vi "Update Room From Server.vi"(8 "error in":errorcluster, 11 "Room Array":refnum<class "Room.lvclass">[](array[class])) -> (0 "error out":errorcluster, 3 "Room Array Out":refnum<class "Room.lvclass">[](array[class]))   [LabVIEW 2015]
uses:
  LVClasses/Room/Room.lvclass
  LVRestAPI/TypeDef/GetRoomCommands.ctl
  LVClasses/Room/Room.lvclass/Room.ctl
  LVRestAPI/RestApi.lvlib
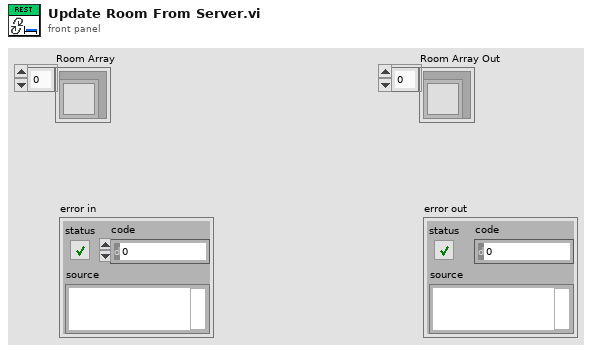
[diagram p1: front panel]
types:
  T1 = typedef "RestApi.lvlib/GetRoomCommands.ctl" = enum16{"ReadRoom", "ReadFlag", "ReadFlagState", "ReadFlagColor", "ReadBedVacant", "ReadPersonnel", "ReadRequests", "ReadBeaconID", "ReadBedURL", "ReadRoomsNumbers"}
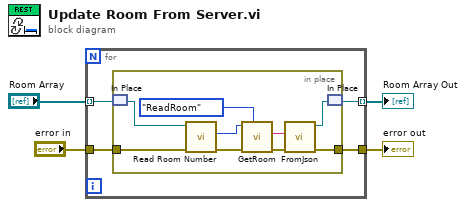
[diagram p0: block diagram]
diagram:
  n1 = for {
    tunnel: "Room Array" -> [w8] mode=indexing
    tunnel: "error in" -> [w7]
    tunnel: [w6] -> w2 mode=indexing
    tunnel: [w5] -> w1
    n2 = in-place {
      in-place-border: w7 -> [w16]
      in-place-border: [w9] -> w5
      n3 = in-place-match #1(w8) -> (w17:refnum<class "Room.lvclass">)
      n4 = call "Read Room Number.vi"("error in (no error)"=w16, "Room in"=w17) -> ("error out"=w15:errorcluster, "Room Number"=w14:i32)  [unwired: 7 in, 1 out]
      n5 = call "GetRoom.vi"("Room Commands"=GetRoomCommands."ReadRoom", "error in (no error)"=w15, "Room Number"=w14) -> ("error out"=w12:errorcluster, "Flags JSON"=w11:string)  [unwired: 7 in]
      n6 = call "FromJson.vi"("error in (no error)"=w12, "String"=w11) -> ("error out"=w9:errorcluster, "Room out"=w10:refnum<class "Room.lvclass">)  [unwired: 8 in]
      n7 = in-place-match #1(w10) -> (w6:refnum<class "Room.lvclass">)
    }
  }
  "Room Array Out" <- w2
  "error out" <- w1
